vi "listandgetdeviceinterface.vi"(10 "error in (no error)":errorcluster, 11 "reference":refnum<k7>) -> (0 "LLTF error out":errorcluster, 1 "LLTFDevice Interface":refnum<k7>, 2 "error out to close":errorcluster, 3 "reference out to lose":refnum<k7>)   [LabVIEW 2019]
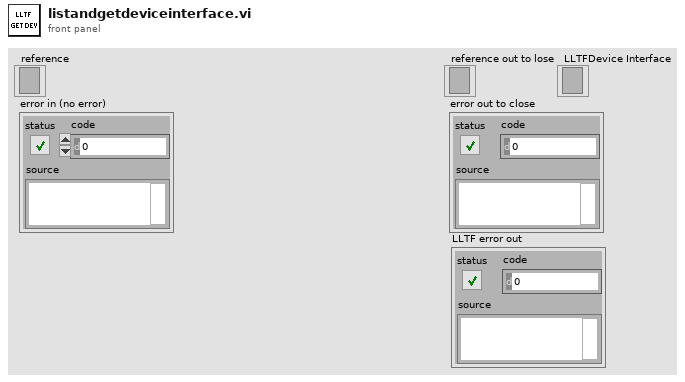
[diagram p1: front panel]
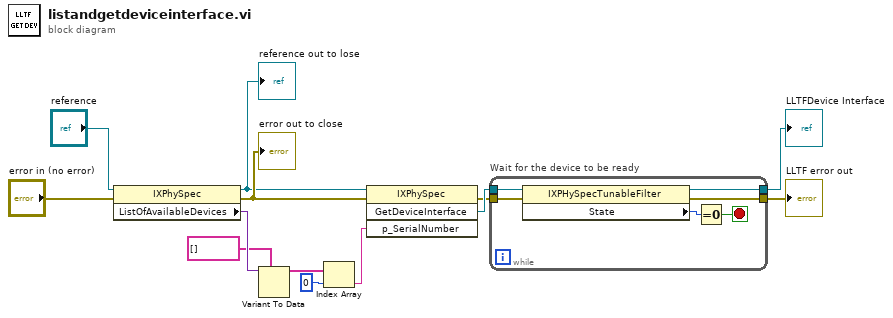
[diagram p0: block diagram]
diagram:
  n1 = property class="IXPhySpec"(reference="reference", error in="error in (no error)") -> (reference out=w12:refnum<k7>, error out=w13:errorcluster, "ListOfAvailableDevices"=w10:variant)
  "reference out to lose" <- w12
  "error out to close" <- w13
  n2 = Variant To Data(type=string[] [], Variant=w10) -> (data=w8:string[])  [unwired: 1 in, 1 out]
  n3 = Index Array(array=w8, index=0) -> (element=w11:string)
  n4 = invoke class="IXPhySpec" method="GetDeviceInterface"(reference=w12, error in=w13, "p_SerialNumber"=w11) -> (error out=w3:errorcluster, "GetDeviceInterface"=w4:refnum<k7>)  [unwired: 1 in, 2 out]
  n5 = while "Wait for the device to be ready" {
    tunnel: [w17] -> w1
    tunnel: w4 -> [w15]
    tunnel: w3 -> [w16]
    tunnel: [w14] -> w2
    stop <- w18 stop-if-true
    n6 = property class="IXPHySpecTunableFilter"(reference=w15, error in=w16) -> (reference out=w14:refnum<k7>, error out=w17:errorcluster, "State"=w19:u32)
    n7 = Equal To 0?(x=w19) -> (x = 0?=w18:bool)
  }
  "LLTFDevice Interface" <- w2
  "LLTF error out" <- w1
